vi "().vi"() -> ()   [LabVIEW 2014]
panel:
  out "Avg. Array":dbl[](array[numeric])
  in  "Array":dbl[][](array[numeric])
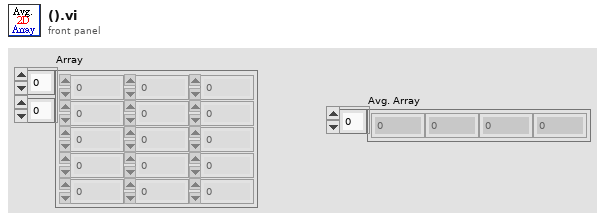
[diagram p1: front panel]
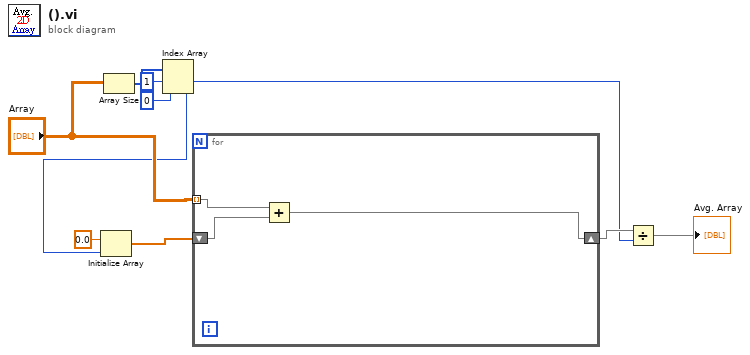
[diagram p0: block diagram]
diagram:
  n1 = Array Size(array="Array") -> (size(s)=w7:i32[])
  n2 = Index Array(array=w7, index #1=1 ("index"), index #2=0 ("index")) -> (element #1=w2:i32, element #2=w4:i32)
  n3 = Initialize Array(0.0 ("element"), w4) -> (w9:dbl[])
  n4 = for {
    shift-right: [w11] -> w3
    shift-left: w9 -> [w13]
    tunnel: "Array" -> [w12] mode=indexing
    n5 = Add(x=w12, y=w13) -> (x+y=w11:dbl[])
  }
  n6 = Divide(x=w3, y=w2) -> (x/y=→"Avg. Array":dbl[])
